vi "ViperHawk Summary Stats.vi"(4 "Cycle Stats":T1, 6 "Day Cycle Count":i32, 9 "Error Code Out":u32, 10 "Time":string, 11 "Date":string) -> (3 "Summary Data":string[](array[string]))   [LabVIEW 2016]
uses:
  Type Definitions/ViperHawk/ViperHawk Summary Stats.ctl
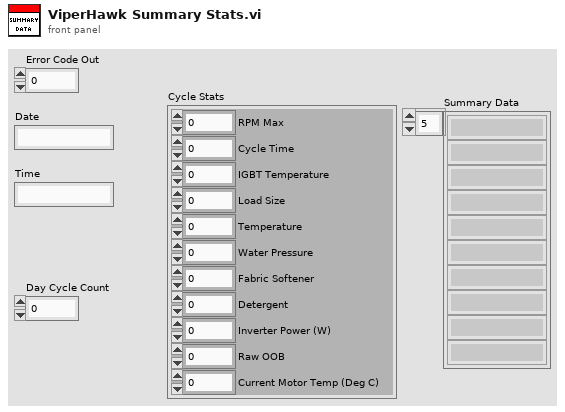
[diagram p1: front panel]
types:
  T1 = typedef "ViperHawk Summary Stats.ctl" = cluster{"RPM Max":u32, "Cycle Time":dbl, "IGBT Temperature":dbl, "Load Size":dbl, "Temperature":dbl, "Water Pressure":dbl, "Detergent":dbl, "Fabric Softener":dbl, "Inverter Power (W)":dbl, "Raw OOB":dbl, "Current Motor Temp (Deg C)":dbl}
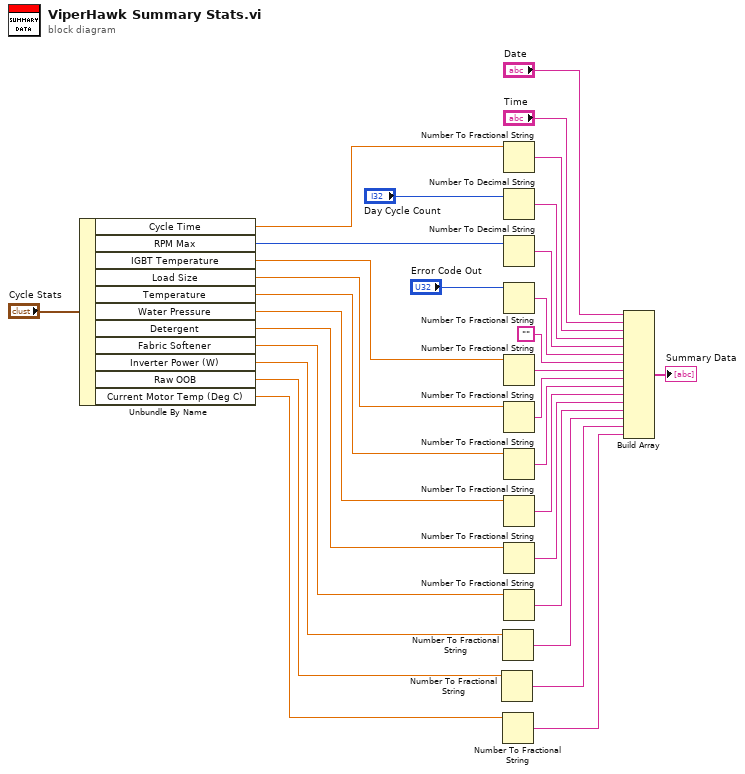
[diagram p0: block diagram]
diagram:
  n1 = Unbundle By Name("Cycle Stats") -> ("Cycle Time"=w21:dbl, "RPM Max"=w20:u32, "IGBT Temperature"=w18:dbl, "Load Size"=w17:dbl, "Temperature"=w16:dbl, "Water Pressure"=w15:dbl, "Detergent"=w14:dbl, "Fabric Softener"=w13:dbl, "Inverter Power (W)"=w6:dbl, "Raw OOB"=w4:dbl, "Current Motor Temp (Deg C)"=w2:dbl)
  n2 = Number To Fractional String(number=w4) -> (F-format string=w3:string)  [unwired: 3 in]
  n3 = Number To Fractional String(number=w6) -> (F-format string=w5:string)  [unwired: 3 in]
  n4 = Number To Fractional String(number=w2) -> (F-format string=w1:string)  [unwired: 3 in]
  n5 = Number To Fractional String(number=w21) -> (F-format string=w28:string)  [unwired: 3 in]
  n6 = Number To Decimal String(number="Day Cycle Count") -> (decimal integer string=w26:string)  [unwired: 1 in]
  n7 = Number To Decimal String(number=w20) -> (decimal integer string=w25:string)  [unwired: 1 in]
  n8 = Number To Fractional String(number="Error Code Out") -> (F-format string=w24:string)  [unwired: 3 in]
  n9 = Number To Fractional String(number=w18) -> (F-format string=w12:string)  [unwired: 3 in]
  n10 = Number To Fractional String(number=w17) -> (F-format string=w11:string)  [unwired: 3 in]
  n11 = Number To Fractional String(number=w16) -> (F-format string=w10:string)  [unwired: 3 in]
  n12 = Number To Fractional String(number=w15) -> (F-format string=w9:string)  [unwired: 3 in]
  n13 = Number To Fractional String(number=w14) -> (F-format string=w8:string)  [unwired: 3 in]
  n14 = Number To Fractional String(number=w13) -> (F-format string=w7:string)  [unwired: 3 in]
  n15 = Build Array("Date", "Time", w28, w26, w25, w24, "", w12, w11, w10, w9, w8, w7, w5, w3, w1) -> (→"Summary Data":string[])
